vi "Size.vi"(8 "error in (no error)":errorcluster, 11 "Time Stamp Array in":refnum<class "Time Stamp Array.lvclass">) -> (0 "error out":errorcluster, 2 "Size":i32, 3 "Time Stamp Array out":refnum<class "Time Stamp Array.lvclass">)   [LabVIEW 2020, in "Data.lvlib" / "Time Stamp Array.lvclass"]
doc: "Return the size of the generic data element."
uses:
  Time Stamp Array.lvclass
  Time Stamp Array.lvclass/Time Stamp Array.ctl
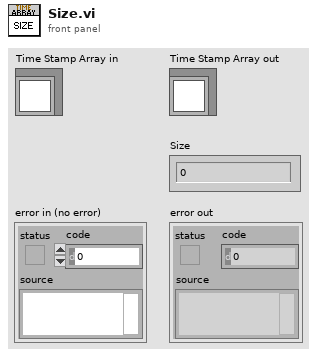
[diagram p1: front panel]
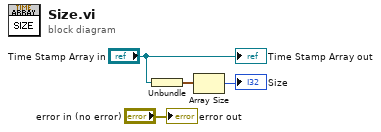
[diagram p0: block diagram]
diagram:
  n1 = Unbundle("Time Stamp Array in") -> (w2:timestamp[])
  n2 = Array Size(array=w2) -> (size(s)=→"Size":i32)
  "error out" <- "error in (no error)"
  "Time Stamp Array out" <- "Time Stamp Array in"
